vi "convertFESTOBytes.vi"(9 "ID Number":u8, 11 "Bytes":u8[](array[numeric])) -> ()   [LabVIEW 2011]
uses:
  GlobalVariables.vi
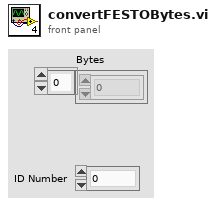
[diagram p1: front panel]
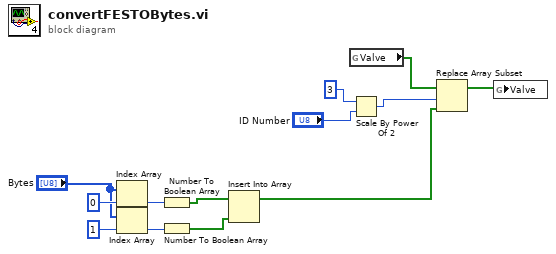
[diagram p0: block diagram]
diagram:
  n1 = Index Array(array="Bytes", index=0) -> (element=w9:u8)
  n2 = Index Array(array="Bytes", index=1) -> (element=w10:u8)
  n3 = Number To Boolean Array(number=w9) -> (Boolean array=w4:bool[])
  n4 = Number To Boolean Array(number=w10) -> (Boolean array=w3:bool[])
  n5 = Insert Into Array(array=w4, new element=w3) -> (w2:bool[])  [unwired: 1 in]
  n6 = global read "GlobalVariables.vi" "Valve"() -> (w8:bool[])
  n7 = Scale By Power Of 2(n=3, x="ID Number") -> (x*2^n=w5:u8)
  n8 = Replace Array Subset(array=w8, new element=w2, index=w5) -> (w1:bool[])
  n9 = global write "GlobalVariables.vi" "Valve"(w1) -> ()
